vi "Waveform_Extract from Start and End TimeStamp with End point.vi"(8 "error in (no error)":errorcluster, 9 "Stop Out":timestamp, 10 "Start Out":timestamp, 11 "Raw Data Waveform":T1) -> (0 "error out":errorcluster, 1 "End Index Out":i32, 2 "Start Index Out":i32, 3 "Waveform Out":T1)   [LabVIEW 2020]
uses:
  Universal Controls/Waveform_Data.ctl
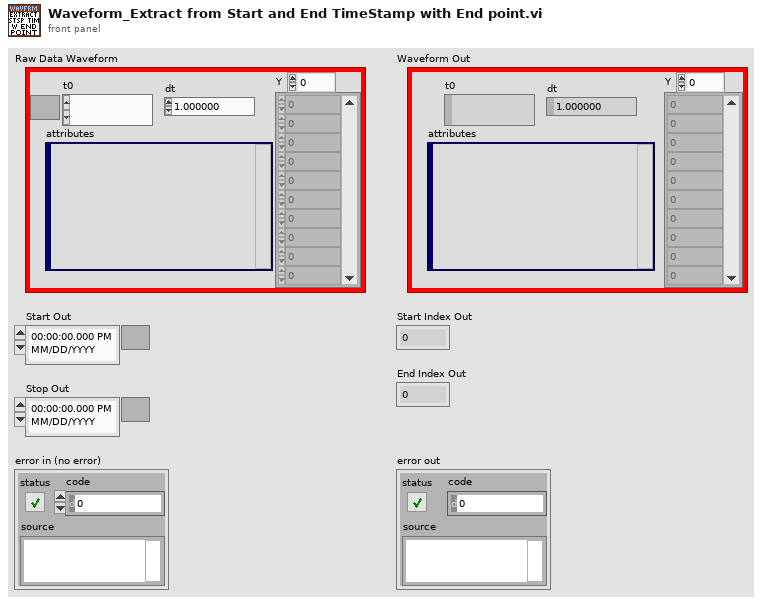
[diagram p1: front panel]
types:
  T1 = typedef "Waveform_Data.ctl" = waveform(dbl)
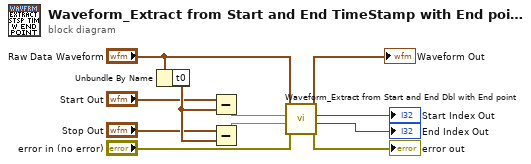
[diagram p0: block diagram]
diagram:
  n1 = Unbundle By Name("Raw Data Waveform") -> ("t0"=w9:timestamp)
  n2 = Subtract(x="Start Out", y=w9) -> (x-y=w10:dbl)
  n3 = Subtract(x="Stop Out", y=w9) -> (x-y=w11:dbl)
  n4 = call "Waveform_Extract from Start and End Dbl with End point.vi"("Error"="error in (no error)", "End Time"=w11, "Begin Time"=w10, "Waveform"="Raw Data Waveform") -> ("Error Out"=→"error out":errorcluster, "End Index Out"=→"End Index Out":i32, "Start Index Out"=→"Start Index Out":i32, "Waveform Out"=→"Waveform Out":T1)  [unwired: 4 in]
